vi "Handle Error.vi"(8 "error in (no error)":errorcluster, 11 "Sim Display Console Actor in":refnum<class "Sim Display Console Actor.lvclass">) -> (0 "error out":errorcluster, 2 "stop actor?":bool=TRUE, 3 "Sim Display Console Actor out":refnum<class "Sim Display Console Actor.lvclass">)   [LabVIEW 2022 SP3, in "Sim Display Console Actor.lvlib" / "Sim Display Console Actor.lvclass"]
doc: "(<B>Filename</B>: Actor Framework.lvlib:Actor.lvclass:Handle Error.vi)\n\nDefines how the actor handles an error that occurred while processing a message.\n\nBy default, this method does nothing except stop the actor. This method also treats error code 43 (coming from <B>error in</B>) as a sign that the actor shut down normally. In this situation, the Handle Error method does not return the error on <B>error out</B>, meaning the actor's caller will not receive it. All other error codes will be returned on <B>error out</B>.\n\nA descendant class may override this method to change this behavior."
uses:
  Sim Display Console Actor.lvclass
  Sim Display Console Actor.lvclass/Sim Display Console Actor.ctl
  Abstract Display Console/Abstract Display Console/Abstract Display Console.lvclass
  Elevator Controller/Elevator Controller Messages/Centralize Error Msg/Centralize Error Msg.lvclass
  <vilib>/ActorFramework/Actor/Actor.lvclass
  C:/Workspace/CLA/Elevator AF_2022/Abstract Display Console/Abstract Display Console/Abstract Display Console.lvclass
  C:/Program Files/National Instruments/LabVIEW 2022/vi.lib/ActorFramework/Actor/Actor.lvclass
  C:/Workspace/CLA/Elevator AF_2022/Sim Display Console Actor/Sim Display Console Actor/Sim Display Console Actor.lvclass
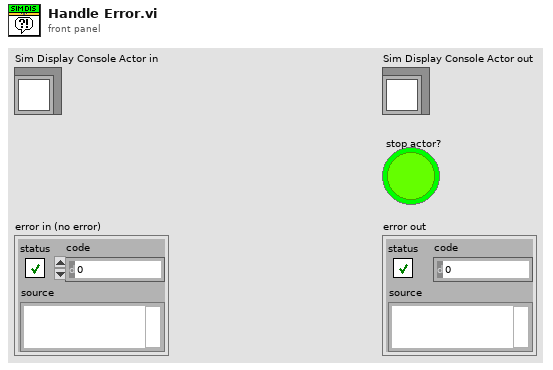
[diagram p1: front panel]
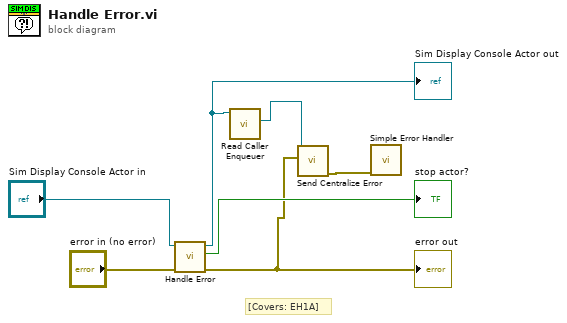
[diagram p0: block diagram]
diagram:
  # "[Covers: EH1A]"
  n1 = call-parent "Handle Error.vi"("error in (no error)"="error in (no error)", "Actor in"="Sim Display Console Actor in") -> ("error out"=w1:errorcluster, "stop actor?"=→"stop actor?":bool, "Actor out"=w2:refnum<class "Sim Display Console Actor.lvclass">)  [unwired: 7 in]
  "Sim Display Console Actor out" <- w2
  "error out" <- w1
  n2 = call <vilib>:"Read Caller Enqueuer.vi"("Actor"=w2) -> ("Caller Enqueuer"=w4:refnum<class "Message Enqueuer.lvclass">)  [unwired: 10 in]
  n3 = call "Send Centralize Error.vi"("Error"=w1, "Message Enqueuer"=w4) -> ("error out"=w3:errorcluster)  [unwired: 8 in, 1 out]
  n4 = call <vilib>:"Simple Error Handler.vi"("error in (no error)"=w3) -> ()  [unwired: 4 in, 5 out]
